vi "Get full path from file name.vi"(1 "File Name":string, 2 "Current Path":path) -> (0 "Full Path":path)   [LabVIEW 2012]
doc: "This subVI returns a full path which points to the file whose name is 'File Name' and it is in the same folder that the current VI."
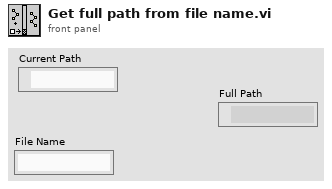
[diagram p1: front panel]
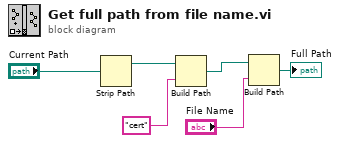
[diagram p0: block diagram]
diagram:
  n1 = Strip Path(path="Current Path") -> (stripped path=w3:path)  [unwired: 1 out]
  n2 = Build Path(base path=w3, name or relative path="cert") -> (appended path=w2:path)
  n3 = Build Path(base path=w2, name or relative path="File Name") -> (appended path=→"Full Path":path)
